vi "BRig_dataTrial_L_Cue_trig_I_l1.vi"() -> (2 "output_L_Cue_trig_I_l1":i32)   [LabVIEW 2014]
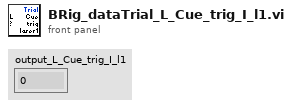
[diagram p1: front panel]
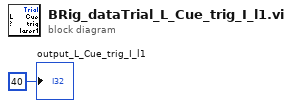
[diagram p0: block diagram]
diagram:
  "output_L_Cue_trig_I_l1" <- 40 ("output_iBlock")
